vi "asset.add_dataset.vi"(8 "error in":errorcluster, 11 "Client in":refnum<class "Client.lvclass">) -> (0 "error out":errorcluster, 3 "Client out":refnum<class "Client.lvclass">)   [LabVIEW 2020, in "Client.lvclass"]
doc: "Attaches a dataset to the asset under the given scope name and returns a handle to the updated asset."
uses:
  Client.lvclass
  client.lvlib
panel:
  out "out_asset out":i32
  in  "rid":string
  in  "scope_name":string
  in  "dataset_rid":string
  in  "out_asset":i32
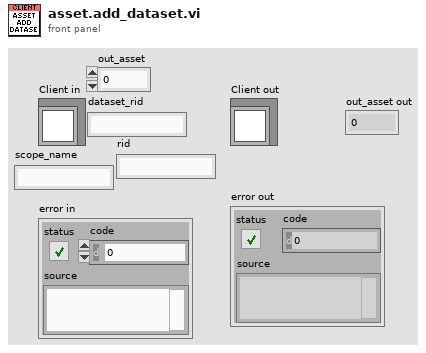
[diagram p1: front panel]
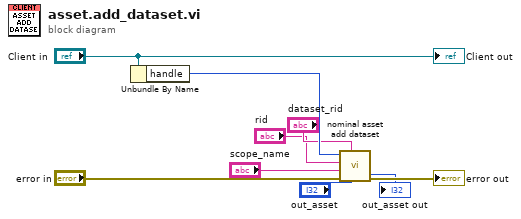
[diagram p0: block diagram]
diagram:
  n1 = Unbundle By Name("Client in") -> ("handle"=w7:i32)
  n2 = call "nominal asset add dataset.vi"("out_asset"="out_asset", "dataset_rid"="dataset_rid", "error in (no error)"="error in", "scope_name"="scope_name", "rid"="rid", "client"=w7) -> ("error out"=→"error out":errorcluster, "out_asset out"=→"out_asset out":i32)  [unwired: 3 in, 1 out]
  "Client out" <- "Client in"
